vi "Control Experiment FGV.vi"(6 "Function":enum16{"read", "write"}(ring), 8 "error in (no error)":errorcluster, 11 "Control Experiment.lvclass":refnum<class "Control Experiment.lvclass">) -> (0 "error out":errorcluster, 3 "Control Experiment.lvclass out":refnum<class "Control Experiment.lvclass">)   [LabVIEW 2019, in "Control Experiment.lvclass"]
uses:
  Control Experiment.lvclass
  <vilib>/Utility/sysdir.llb/System Directory Type.ctl
  Control Experiment.lvclass/Control Experiment.ctl
  <vilib>/Utility/xml.llb/Write to XML File(string).vi
  <vilib>/Utility/xml.llb/Read From XML File(string).vi
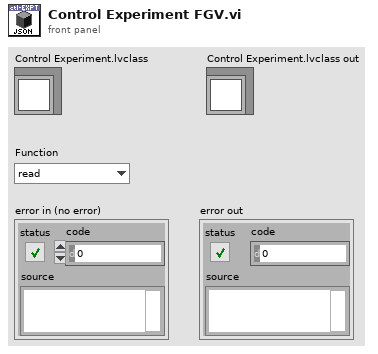
[diagram p1: front panel]
types:
  T1 = typedef "System Directory Type.ctl" = i32
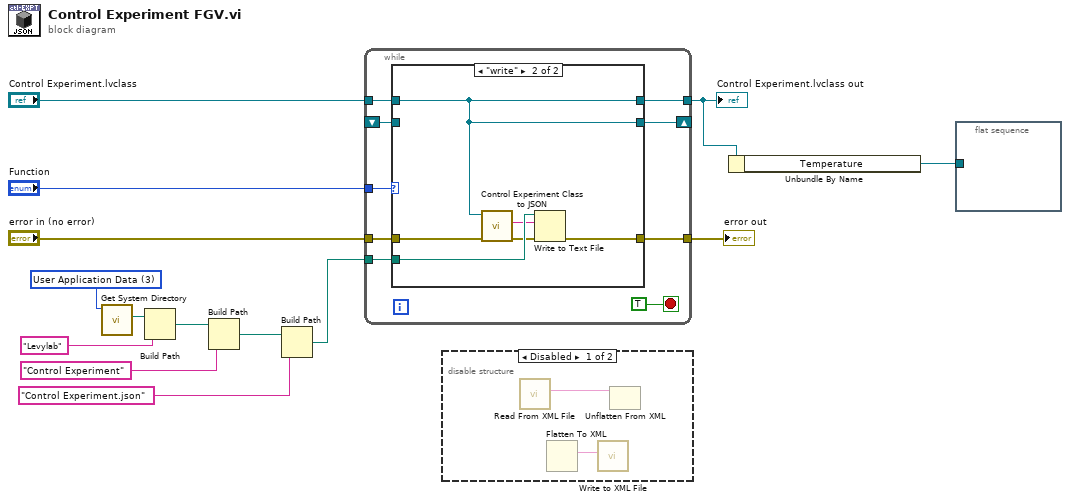
[diagram p0: block diagram]
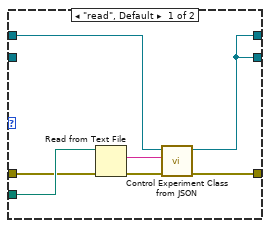
[diagram p3: hidden frame]
diagram:
  w9 = T1 3 items=["User Home"=0, "User Desktop"=1, "User Documents"=2, "User Application Data"=3, "User Preferences"=4, "User Temporary"=5, "Public Documents"=6, "Public Application Data"=7, "Public Preferences"=8, "Public Cache"=13, "System Core Libraries"=9, "System Installed Libraries"=10, "Application Files"=11, "Boot Volume Root"=12] ("system directory type")
  n1 = call <vilib>:"Get System Directory.vi"("system directory type"=w9) -> ("system directory"=w6:path)  [unwired: 10 in]
  n2 = Build Path(base path=w6, name or relative path="Levylab") -> (appended path=w8:path)
  n3 = Build Path(base path=w8, name or relative path="Control Experiment") -> (appended path=w3:path)
  n4 = Build Path(base path=w3, name or relative path="Control Experiment.json") -> (appended path=w4:path)
  n5 = while {
    tunnel: "Control Experiment.lvclass" -> [w20]
    tunnel: "error in (no error)" -> [w17]
    tunnel: [w16] -> w14
    tunnel: [w19] -> w2
    shift-right: [w21] -> _
    shift-left: _ -> [w18]
    tunnel: "Function" -> [w22]
    tunnel: w4 -> [w15]
    stop <- TRUE stop-if-true
    n6 = case shown="\"write\"" w22 {
      tunnel: [w29 w32] -> w21
      tunnel: w20 -> [w25 w32]
      tunnel: [w29 w32] -> w19
      tunnel: w18 -> [_ _]
      tunnel: w17 -> [w24 w33]
      tunnel: [w30 w35] -> w16
      tunnel: w15 -> [w28 w36]
      frame "read", Default {
        n7 = Read from Text File(file (use dialog)=w28, error in=w24) -> (text=w27:string, error out=w26:errorcluster)  [unwired: 2 in, 2 out]
        n8 = call "Control Experiment Class from JSON.vi"("error in (no error)"=w26, "JSON"=w27, "Control Experiment in"=w25) -> ("error out"=w30:errorcluster, "Control Experiment out"=w29:refnum<class "Control Experiment.lvclass">)  [unwired: 7 in]
      }
      frame "write" {
        n9 = call "Control Experiment Class to JSON.vi"("error in (no error)"=w33, "Control Experiment in"=w32) -> ("error out"=w34:errorcluster, "<JSON>"=w31:string)  [unwired: 7 in, 1 out]
        n10 = Write to Text File(file (use dialog)=w36, text=w31, error in=w34) -> (error out=w35:errorcluster)  [unwired: 1 in, 2 out]
      }
    }
  }
  "error out" <- w14
  "Control Experiment.lvclass out" <- w2
  n11 = disable-structure shown="Disabled" {
    frame Disabled {
      n12 = call-poly <vilib>:"Read From XML File.vi"() -> ("XML Elements"=w38:string)  [unwired: 9 in, 2 out]
      n13 = Flatten To XML() -> (xml string=w39:string)  [unwired: 1 in]
      n14 = call-poly <vilib>:"Write to XML File.vi"("XML Input"=w39) -> ()  [unwired: 8 in, 3 out]
      n15 = Unflatten From XML(xml string=w38) -> (type=w37:cluster{})  [unwired: 1 in, 2 out]
    }
    frame Enabled {
    }
  }
  n16 = Unbundle By Name(w2) -> ("Temperature"=w1:refnum<class "Instrument.Cryostat.lvclass">)
  n17 = flat-sequence {
    tunnel: w1 -> [_]
    frame #0 {
    }
  }
